vi "init.vi"(8 "error in (no error)":errorcluster, 11 "Logger in":refnum<class "TestDataLog.lvclass">) -> (0 "error out":errorcluster, 3 "Logger out":refnum<class "TestDataLog.lvclass">)   [LabVIEW 2015, in "TestDataLog.lvclass"]
uses:
  TestDataLog.lvclass
  Configuration/SystemController.ctl
  <userlib>/Common/Log/Config/Log.ctl
  StiffnessCalculator/Preconditioning.ctl
  TestDataLog.lvclass/TestDataLog.ctl
  <userlib>/Common/Log/Log/Log.lvclass/Log.ctl
  ConfigurationThisComponent/ConfigurationThisComponent.lvclass
  <userlib>/Common/Log/Log/Log.lvclass
  <userlib>/Common/Log/Log.lvlib
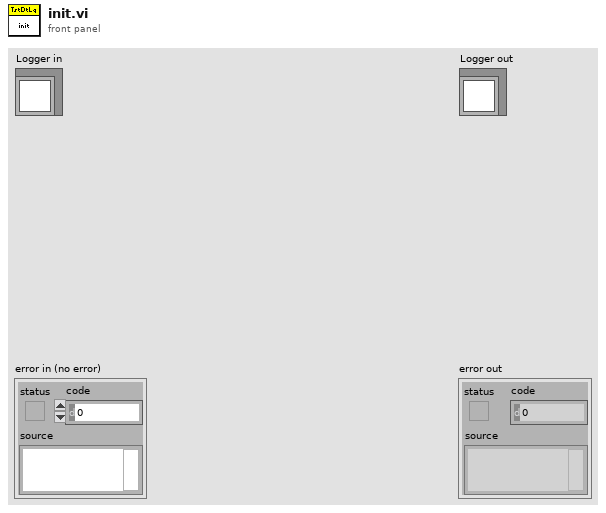
[diagram p1: front panel]
types:
  T1 = typedef "Preconditioning.ctl" = cluster{"Number of Preconditioning Cycles":u32}
  T2 = typedef "Log.lvlib/Log.ctl" = cluster{"Log Directory":path, "Log Filename Base":string, "Max records per file":u32, "Comment":string, "DUT ID":string}
  T3 = typedef "SystemController.ctl" = cluster{"PreconditioningRamp Rate (%/s)":dbl[unit], "Stiffness Test Ramp Rate (%/s)":dbl[unit], "Preconditioning Ramp Target":cluster{"Displacement":dbl[unit]}, "Stiffness Test Ramp Targets":cluster{"Displacement":dbl[unit], "Target Force":dbl[unit]}, "Settling":cluster{"Displacement Max StDev":dbl[unit], "Evaluation Time":dbl[unit]}}
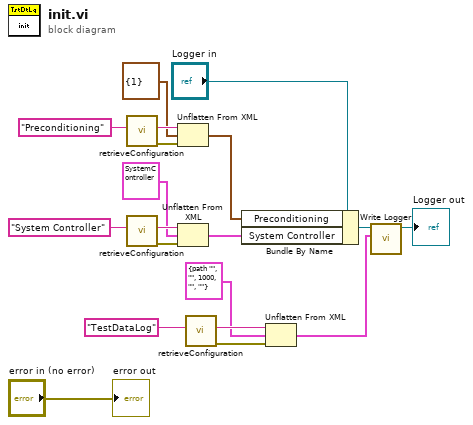
[diagram p0: block diagram]
diagram:
  n1 = call "retrieveConfiguration.vi"("configName"="Preconditioning") -> ("error out"=w4:errorcluster, "xmlConfig"=w3:string)  [unwired: 8 in, 1 out]
  n2 = call "retrieveConfiguration.vi"("configName"="System Controller") -> ("error out"=w17:errorcluster, "xmlConfig"=w16:string)  [unwired: 8 in, 1 out]
  n3 = Unflatten From XML(xml string=w3, type=T1 {"Number of Preconditioning Cycles"=1} ("Preconditioning"), error in (no error)=w4) -> (value=w1:T1)  [unwired: 1 out]
  n4 = Unflatten From XML(xml string=w16, type=T3 {"PreconditioningRamp Rate (%/s)"=2.0, "Stiffness Test Ramp Rate (%/s)"=2.0, "Preconditioning Ramp Target"={"Displacement"=2e-06}, "Stiffness Test Ramp Targets"={"Displacement"=2e-06, "Target Force"=8.896444}, "Settling"={"Displacement Max StDev"=2e-06, "Evaluation Time"=2.0}} ("System Controller"), error in (no error)=w17) -> (value=w14:T3)  [unwired: 1 out]
  n5 = call "retrieveConfiguration.vi"("configName"="TestDataLog") -> ("error out"=w11:errorcluster, "xmlConfig"=w12:string)  [unwired: 8 in, 1 out]
  n6 = Bundle By Name(cluster="Logger in", "Preconditioning"=w1, "System Controller"=w14) -> (w9:refnum<class "TestDataLog.lvclass">)
  n7 = Unflatten From XML(xml string=w12, type=T2 {"Log Directory"=path "", "Log Filename Base"="", "Max records per file"=1000, "Comment"="", "DUT ID"=""} ("Logger"), error in (no error)=w11) -> (value=w7:T2)  [unwired: 1 out]
  n8 = call <userlib>:"Write Logger.vi"("Logger"=w7, "Logger in"=w9) -> ("Logger out"=→"Logger out":refnum<class "TestDataLog.lvclass">)  [unwired: 9 in]
  "error out" <- "error in (no error)"
